vi "Proportional Stepper.vi"(0 "frontLeftNow":dbl, 1 "frontLeftPrev":dbl, 2 "frontRightNow":dbl, 3 "frontRightPrev":dbl, 4 "rearLeftNow":dbl, 5 "rearLeftPrev":dbl, 6 "rearRightNow":dbl, 7 "rearRightPrev":dbl, 11 "Limit":dbl) -> (21 "frontLeft'":dbl, 23 "frontRight'":dbl, 25 "rearLeft'":dbl, 27 "rearRight'":dbl)   [LabVIEW 2013]
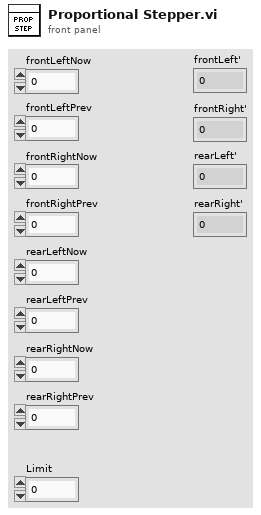
[diagram p1: front panel]
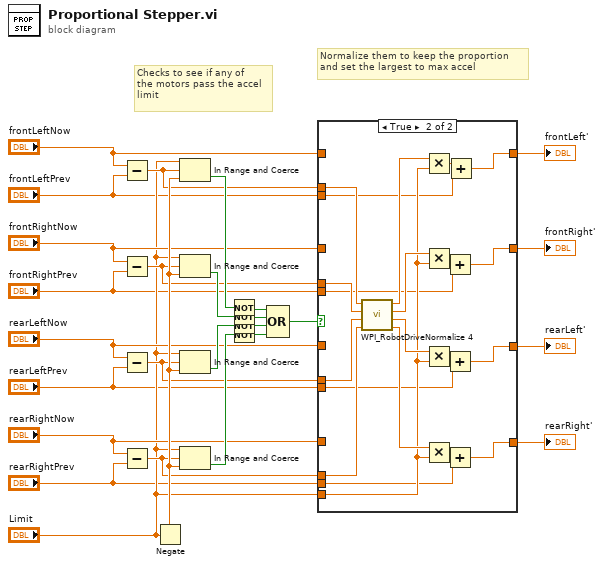
[diagram p0: block diagram]
diagram:
  # "Normalize them to keep the proportion\nand set the largest to max accel"
  # "Checks to see if any of \nthe motors pass the accel\nlimit"
  n1 = Subtract(x="frontLeftNow", y="frontLeftPrev") -> (x-y=w10:dbl)
  n2 = Subtract(x="frontRightNow", y="frontRightPrev") -> (x-y=w9:dbl)
  n3 = Subtract(x="rearLeftNow", y="rearLeftPrev") -> (x-y=w8:dbl)
  n4 = Subtract(x="rearRightNow", y="rearRightPrev") -> (x-y=w7:dbl)
  n5 = Negate(x="Limit") -> (-x=w27:dbl)
  n6 = In Range and Coerce(upper limit="Limit", x=w10, lower limit=w27) -> (In Range?=w26:bool)  [unwired: 1 out]
  n7 = In Range and Coerce(upper limit="Limit", x=w9, lower limit=w27) -> (In Range?=w23:bool)  [unwired: 1 out]
  n8 = In Range and Coerce(upper limit="Limit", x=w8, lower limit=w27) -> (In Range?=w24:bool)  [unwired: 1 out]
  n9 = In Range and Coerce(upper limit="Limit", x=w7, lower limit=w27) -> (In Range?=w25:bool)  [unwired: 1 out]
  n10 = Not(x=w26) -> (.not. x?=w19:bool)
  n11 = Not(x=w23) -> (.not. x?=w20:bool)
  n12 = Not(x=w24) -> (.not. x?=w21:bool)
  n13 = Not(x=w25) -> (.not. x?=w22:bool)
  n14 = Compound Arithmetic op=OR(w19, w20, w21, w22) -> (w18:bool)
  n15 = case shown="True" w18 {
    tunnel: "rearRightNow" -> [w28 _]
    tunnel: "rearLeftNow" -> [w29 _]
    tunnel: "frontRightNow" -> [w30 _]
    tunnel: "frontLeftNow" -> [w31 _]
    tunnel: [w31 w32] -> w11
    tunnel: [w30 w33] -> w12
    tunnel: [w29 w48] -> w13
    tunnel: [w28 w47] -> w14
    tunnel: w10 -> [_ w52]
    tunnel: w9 -> [_ w51]
    tunnel: w8 -> [_ w50]
    tunnel: w7 -> [_ w49]
    tunnel: "Limit" -> [_ w42]
    tunnel: "frontLeftPrev" -> [_ w41]
    tunnel: "frontRightPrev" -> [_ w34]
    tunnel: "rearLeftPrev" -> [_ w35]
    tunnel: "rearRightPrev" -> [_ w36]
    frame False {
      # "All within range"
    }
    frame True {
      n16 = call <vilib>:"WPI_RobotDriveNormalize 4.vi"("D"=w49, "C"=w50, "B"=w51, "A"=w52) -> ("D'"=w43:dbl, "C'"=w44:dbl, "B'"=w45:dbl, "A'"=w46:dbl)
      n17 = Multiply(x=w46, y=w42) -> (x*y=w40:dbl)
      n18 = Multiply(x=w45, y=w42) -> (x*y=w39:dbl)
      n19 = Multiply(x=w44, y=w42) -> (x*y=w38:dbl)
      n20 = Multiply(x=w43, y=w42) -> (x*y=w37:dbl)
      n21 = Add(x=w39, y=w34) -> (x+y=w33:dbl)
      n22 = Add(x=w38, y=w35) -> (x+y=w48:dbl)
      n23 = Add(x=w37, y=w36) -> (x+y=w47:dbl)
      n24 = Add(x=w40, y=w41) -> (x+y=w32:dbl)
    }
  }
  "frontLeft'" <- w11
  "frontRight'" <- w12
  "rearLeft'" <- w13
  "rearRight'" <- w14
